vi "testEXT Data Arrays Failure With Location In Message.vi"(8 "error in (no error)":errorcluster, 11 "TestCase in":refnum<class "1D Array Test Case.lvclass">) -> (0 "error out":errorcluster, 3 "TestCase out":refnum<class "1D Array Test Case.lvclass">)   [LabVIEW 2015, in "1D Array Test Case.lvclass"]
uses:
  1D Array Test Case.lvclass
  <vilib>/addons/_JKI Toolkits/VI Tester/TestCase.llb/TestCase.lvclass
  VITAC.lvlib
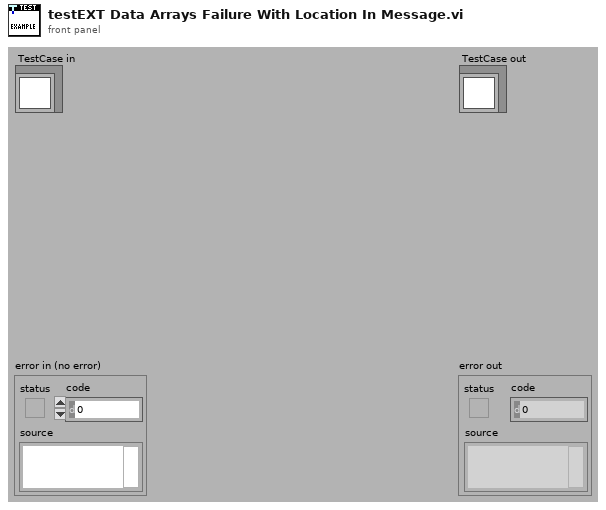
[diagram p1: front panel]
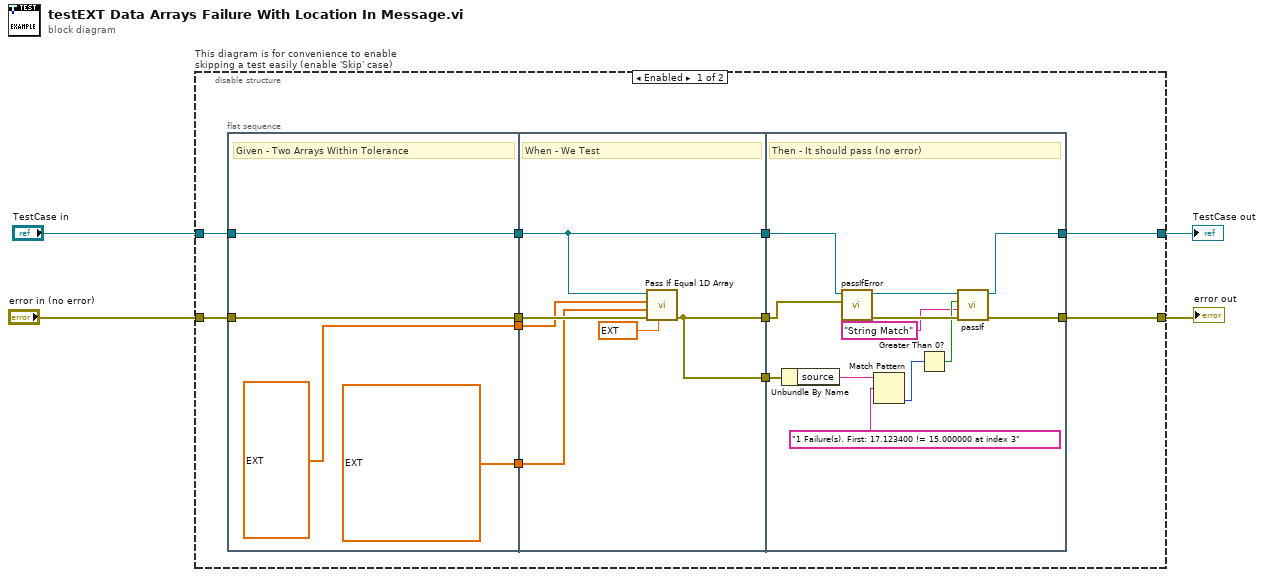
[diagram p0: block diagram]
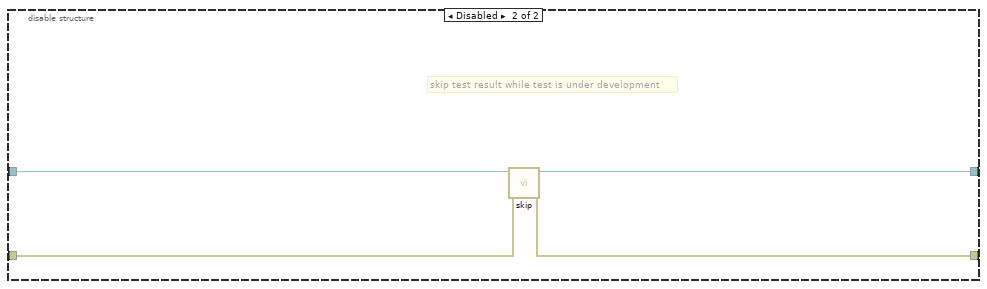
[diagram p2: hidden frame]
diagram:
  n1 = disable-structure "This diagram is for convenience to enable skipping a test easily (enable 'Skip' case)" shown="Enabled" {
    disable-tunnel: "TestCase in" -> [w14 w41]
    disable-tunnel: [w13 w39] -> w1
    disable-tunnel: [w10 w40] -> w3
    disable-tunnel: "error in (no error)" -> [w11 w38]
    frame Enabled {
      n2 = flat-sequence {
        tunnel: [w19] -> w15
        tunnel: w14 -> [w19]
        tunnel: [w18] -> w12
        tunnel: w11 -> [w18]
        tunnel: [ext[] [12.0, 13.0, 14.0, 15.0, 16.0, 17.0, 20000000000.0] ("x")] -> w8
        tunnel: [ext[] [12.0004999999999999996, 13.0, 14.0004999999999999996, 17.123399999999999999, 16.0, 17.0, 20000000000.0] ("x")] -> w7
        tunnel: w15 -> [w21]
        tunnel: w12 -> [w25]
        tunnel: [w20] -> w9
        tunnel: w8 -> [w23]
        tunnel: w7 -> [w22]
        tunnel: [w21] -> w6
        tunnel: [w20] -> w5
        tunnel: [w32] -> w13
        tunnel: [w34] -> w10
        tunnel: w9 -> [w35]
        tunnel: w6 -> [w36]
        tunnel: w5 -> [w31]
        frame #0 {
          # "Given - Two Arrays Within Tolerance"
        }
        frame #1 {
          # "When - We Test"
          n3 = call "Pass If Equal 1D Array.vi"("delta (optional)"=ext 0.0006, "error in (no error)"=w25, "actual"=w22, "expected"=w23, "TestCase in"=w21) -> ("error out"=w20:errorcluster)  [unwired: 5 in, 1 out]
        }
        frame #2 {
          # "Then - It should pass (no error)"
          n4 = Unbundle By Name(w31) -> ("source"=w30:string)
          n5 = call-dynamic "passIfError.vi"("error"=w35, "TestCase in"=w36) -> ("error out"=w37:errorcluster, "TestCase out"=w33:refnum<class "1D Array Test Case.lvclass">)  [unwired: 8 in]
          n6 = Match Pattern(string=w30, regular expression="1 Failure(s). First: 17.123400 != 15.000000 at index 3") -> (offset past match=w28:i32)  [unwired: 1 in, 3 out]
          n7 = Greater Than 0?(x=w28) -> (x > 0?=w27:bool)
          n8 = call-dynamic "passIf.vi"("error in (no error)"=w37, "message (\"\")"="String Match" ("message (\"\")"), "pass"=w27, "TestCase in"=w33) -> ("error out"=w34:errorcluster, "TestCase out"=w32:refnum<class "1D Array Test Case.lvclass">)  [unwired: 6 in]
        }
      }
    }
    frame Disabled {
      # "skip test result while test is under development"
      n9 = call <vilib>:"skip.vi"("error in (no error)"=w38, "TestCase in"=w41) -> ("error out"=w40:errorcluster, "TestCase out"=w39:refnum<class "1D Array Test Case.lvclass">)  [unwired: 8 in]
    }
  }
  "error out" <- w3
  "TestCase out" <- w1
